vi "Sort by Elem ArrCl.vi"(8 "Objects In":T1[](array[typedef]) {"Aspect Ratio" format="%.2f"; "Orientation" format="%.2f"; "Area" format="%.2f"; "Object Center"."Y" format="%.2f"; "Object Center"."X" format="%.2f"}) -> (0 "Objects Out":T1[](array[typedef]) {"Aspect Ratio" format="%.2f"; "Orientation" format="%.2f"; "Area" format="%.2f"; "Object Center"."Y" format="%.2f"; "Object Center"."X" format="%.2f"})   [LabVIEW 2015]
uses:
  TypeDefs Host/Object Info.ctl
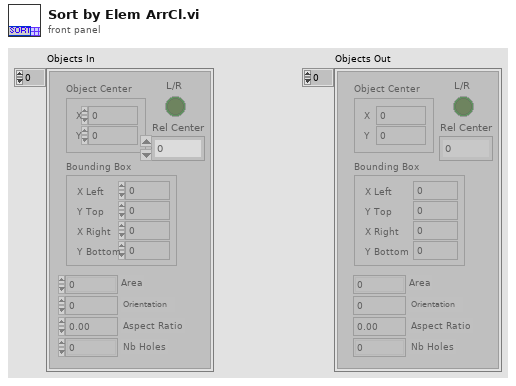
[diagram p1: front panel]
types:
  T1 = typedef "Object Info.ctl" = cluster{"Object Center":cluster{"X":u16, "Y":u16}, "Bounding Box":cluster{"X Left":u16, "Y Top":u16, "X Right":u16, "Y Bottom":u16}, "Area":u16, "Orientation":u16, "Aspect Ratio":sgl, "Nb Holes":u16, "L/R":bool, "Rel Center":u16}
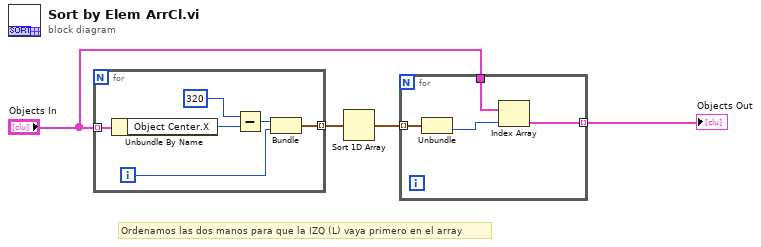
[diagram p0: block diagram]
diagram:
  # "Ordenamos las dos manos para que la IZQ (L) vaya primero en el array"
  n1 = for {
    tunnel: "Objects In" -> [w10] mode=indexing
    tunnel: [w8] -> w4 mode=indexing
    i -> [w9]
    n2 = Unbundle By Name(w10) -> ("Object Center.X"=w5:u16)
    n3 = Subtract(x=u16 320 ("Object Center.X"), y=w5) -> (x-y=w7:u16)
    n4 = Bundle(w7, w9) -> (w8:cluster{u16, i32})  [unwired: 1 in]
  }
  n5 = Sort 1D Array(array=w4) -> (sorted array=w3:cluster{u16, i32}[])
  n6 = for {
    tunnel: w3 -> [w14] mode=indexing
    tunnel: "Objects In" -> [w12]
    tunnel: [w11] -> w1 mode=indexing
    n7 = Unbundle(w14) -> (w13:i32)  [unwired: 1 out]
    n8 = Index Array(array=w12, index=w13) -> (element=w11:T1)
  }
  "Objects Out" <- w1
